vi "Handle Command.vi"(8 "error in (no error)":errorcluster, 9 "Data":variant, 10 "Command":string, 11 "LakeShore.340 in":refnum<class "LakeShore.340.lvclass">) -> (0 "error out":errorcluster, 1 "Processed Data":variant, 2 "Command":string, 3 "LakeShore.340 out":refnum<class "LakeShore.340.lvclass">)   [LabVIEW 2016, in "LakeShore.340.lvclass"]
uses:
  LakeShore.340.lvclass
  <userlib>/LevyLab/Levylab Instruments/SMOs/Instrument/Instrument.lvclass
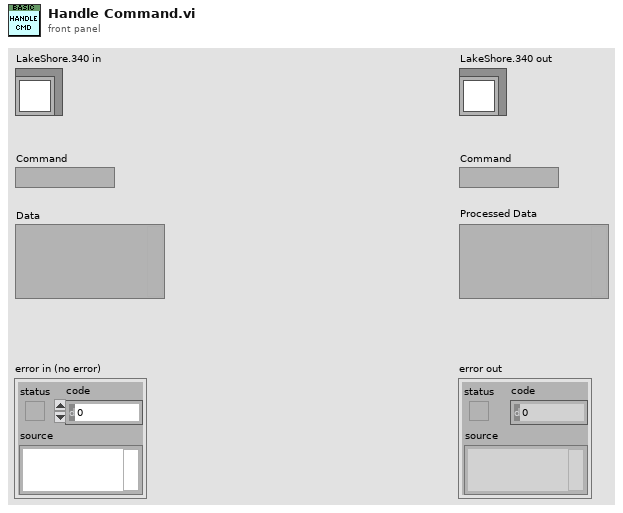
[diagram p1: front panel]
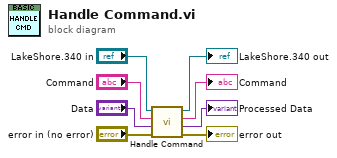
[diagram p0: block diagram]
diagram:
  n1 = call-parent "Handle Command.vi"("error in (no error)"="error in (no error)", "Data"="Data", "Command"="Command", "Instrument in"="LakeShore.340 in") -> ("error out"=→"error out":errorcluster, "Processed Data"=→"Processed Data":variant, "Command"=→"Command":string, "Instrument out"=→"LakeShore.340 out":refnum<class "LakeShore.340.lvclass">)  [unwired: 4 in]
